vi "Config Process.vi"(8 "error in (no error)":errorcluster, 11 "View Model":T3) -> (0 "error out":errorcluster)   [LabVIEW 2017]
doc: "Configuration DB Process provide full access to the data records\nand process requests from controller\n[Covers: SD6]"
uses:
  Model/Controls/View Model.ctl
  Model/Controls/Shared Model.ctl
  Model/Controls/Views Action.ctl
  Error Handler/Controls/Error Model.ctl
  Error Handler/Controls/Error Message.ctl
  Error Handler/Controls/Error Type.ctl
  Controls/Config Model.ctl
  Controls/Config DB Message.ctl
  Controls/Config DB Command.ctl
  Controls/Config DB Overhead.ctl
  Controls/Config DB Record.ctl
  Controller/Controls/Controller Model.ctl
  Views/Vehicle Position Simulation View/Controls/Vehicle - Position.ctl
  Controller/Controls/Controller Overhead.ctl
  Controller/Controls/Controller Wash Step.ctl
  Controller/Controls/Controller State.ctl
panel:
  in  "Execute":bool
  out "Config DB Records Array":T1[](array[typedef])
  in  "DB Record":T1
  in  "DB Command":T2
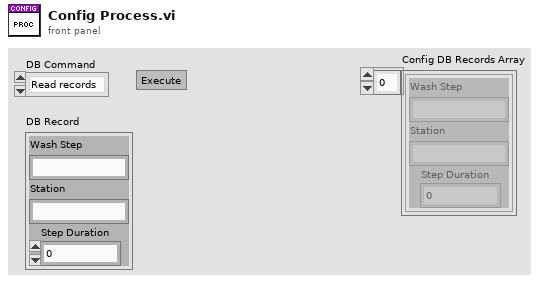
[diagram p1: front panel]
types:
  T1 = typedef "Config DB Record.ctl" = cluster{"Wash Step":string, "Station":string, "Step Duration":u32}
  T2 = typedef "Config DB Command.ctl" = enum16{"Read records", "Query timing", "Insert new data", "Update data", "Lock DB", "Unlock DB"}
  T3 = typedef "View Model.ctl" = cluster{"Shared Model":T4, "Error Model":T5, "Config Model":T6, "Controller Model":T7}
  T4 = typedef "Shared Model.ctl" = cluster{"Stop":refnum<user-event>, "Stop DVR":refnum<data-value>, "Views Action":refnum<user-event>}
  T5 = typedef "Error Model.ctl" = cluster{"Error":refnum<user-event>}
  T6 = typedef "Config Model.ctl" = cluster{"Config":refnum<user-event>, "Config DVR":refnum<data-value>}
  T7 = typedef "Controller Model.ctl" = cluster{"Position Change":refnum<user-event>, "Overhead DVR":refnum<data-value>, "Wash Cycle Start":refnum<user-event>, "Wash Step Start":refnum<user-event>, "Out Of Position":refnum<user-event>}
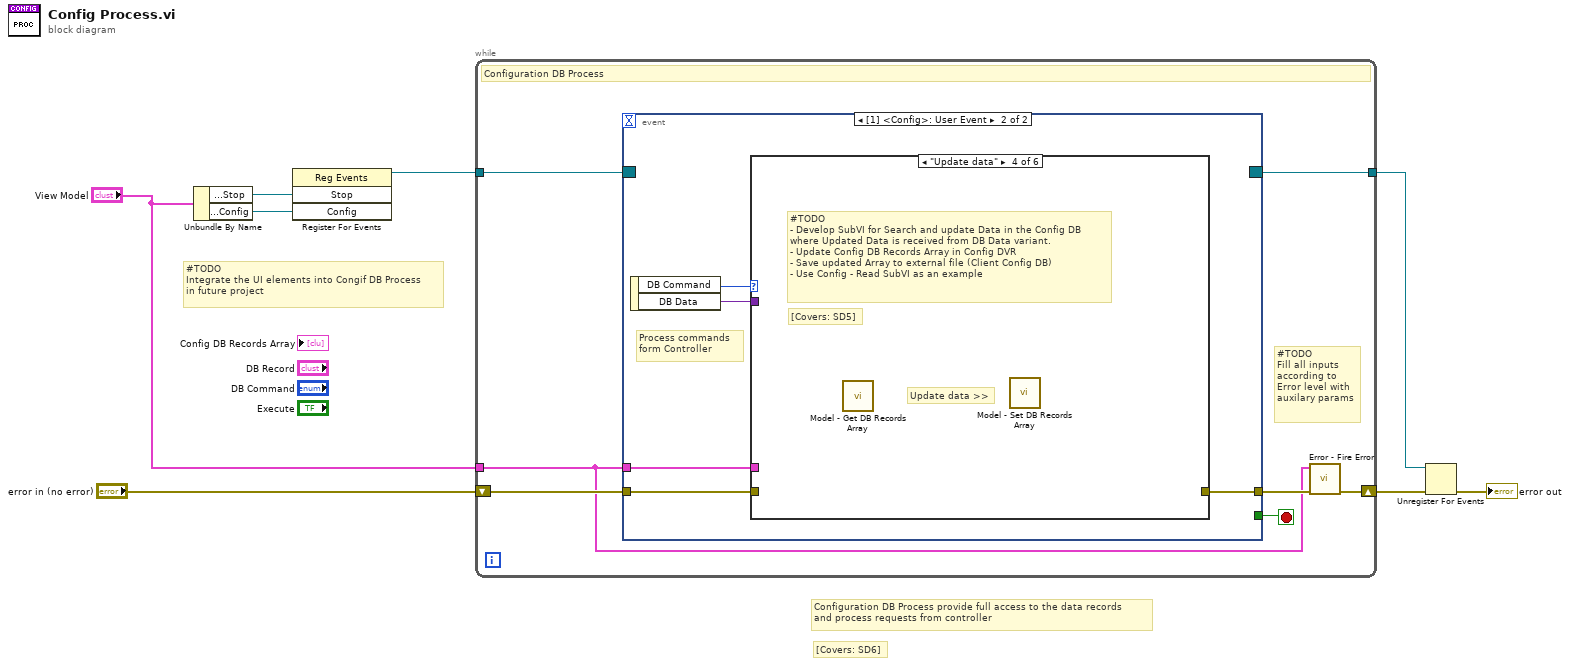
[diagram p0: block diagram]
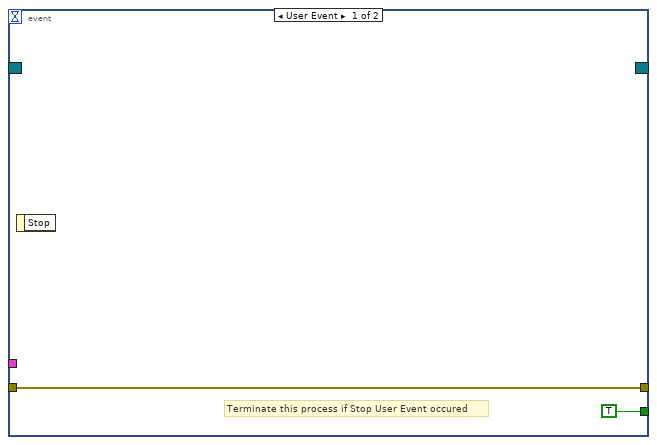
[diagram p2: hidden frame]
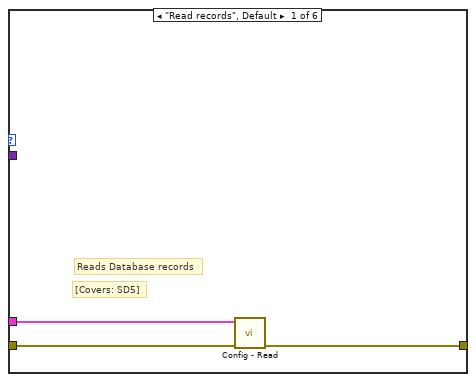
[diagram p3: hidden frame]
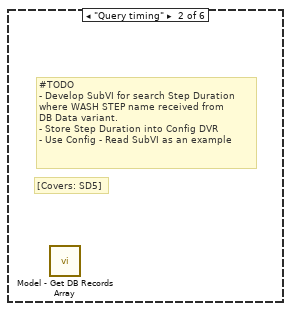
[diagram p4: hidden frame]
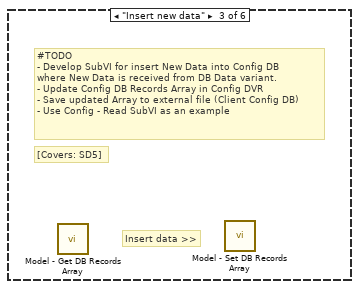
[diagram p5: hidden frame]
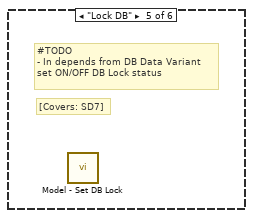
[diagram p6: hidden frame]
diagram:
  # "#TODO\nIntegrate the UI elements into Congif DB Process\nin future project"
  # "[Covers: SD6]"
  # "Configuration DB Process provide full access to the data records\nand process requests from controller"
  n1 = Unbundle By Name("View Model") -> ("Shared Model.Stop"=w8:refnum<user-event>, "Config Model.Config"=w1:refnum<user-event>)
  n2 = register-events(w8, w1) -> (reference out=w7:refnum<event-registration>)  [unwired: 2 in, 1 out]
  n3 = while {
    tunnel: w7 -> [w15]
    shift-right: [w10] -> w5
    shift-left: "error in (no error)" -> [w14]
    tunnel: [w13] -> w3
    tunnel: "View Model" -> [w9]
    stop <- w12 stop-if-true
    # "#TODO\nFill all inputs\naccording to \nError level with\nauxilary params"
    # "Configuration DB Process"
    n4 = event shown="[1] <Config>: User Event" {
      selector: w15 -> [_ _]
      dyn-events: [_ _] -> w13
      timeout: _ -> [_ _]
      tunnel: w14 -> [w17 w20]
      tunnel: [w17 w19] -> w11
      tunnel: w9 -> [_ w21]
      tunnel: [TRUE _] -> w12
      event User Event {
        # "Terminate this process if Stop User Event occured"
        n5 = event-data() -> ()  [unwired: 1 in, 1 out]
      }
      event User Event {
        # "Process commands\nform Controller"
        n6 = event-data() -> ("DB Command"=w22:T2, "DB Data"=w18:variant)  [unwired: 1 in]
        n7 = case shown="\"Update data\"" w22 {
          tunnel: w21 -> [w25 _ _ _ _ _]
          tunnel: w20 -> [w24 _ _ _ _ _]
          tunnel: [w23 _ _ _ _ _] -> w19
          tunnel: w18 -> [_ _ _ _ _ _]
          frame "Read records", Default {
            # "[Covers: SD5]"
            # "Reads Database records"
            n8 = call "Config - Read.vi"("error in (no error)"=w24, "View Model"=w25) -> ("error out"=w23:errorcluster)  [unwired: 8 in, 1 out]
          }
          frame "Query timing" {
            # "[Covers: SD5]"
            # "#TODO\n- Develop SubVI for search Step Duration\nwhere WASH STEP name received from\nDB Data variant.\n- Store Step Duration into Config DVR\n- Use Config - Read SubVI as an example"
            n9 = call "Model - Get DB Records Array.vi"() -> ()  [unwired: 9 in, 3 out]
          }
          frame "Insert new data" {
            # "Insert data >>"
            # "[Covers: SD5]"
            # "#TODO\n- Develop SubVI for insert New Data into Config DB\nwhere New Data is received from DB Data variant.\n- Update Config DB Records Array in Config DVR\n- Save updated Array to external file (Client Config DB)\n- Use Config - Read SubVI as an example"
            n10 = call "Model - Get DB Records Array.vi"() -> ()  [unwired: 9 in, 3 out]
            n11 = call "Model - Set DB Records Array.vi"() -> ()  [unwired: 10 in, 2 out]
          }
          frame "Update data" {
            # "Update data >>"
            # "[Covers: SD5]"
            # "#TODO\n- Develop SubVI for Search and update Data in the Config DB\nwhere Updated Data is received from DB Data variant.\n- Update Config DB Records Array in Config DVR\n- Save updated Array to external file (Client Config DB)\n- Use Config - Read SubVI as an example"
            n12 = call "Model - Get DB Records Array.vi"() -> ()  [unwired: 9 in, 3 out]
            n13 = call "Model - Set DB Records Array.vi"() -> ()  [unwired: 10 in, 2 out]
          }
          frame "Lock DB" {
            # "[Covers: SD7]"
            # "#TODO\n- In depends from DB Data Variant\nset ON/OFF DB Lock status"
            n14 = call "Model - Set DB Lock.vi"() -> ()  [unwired: 10 in, 2 out]
          }
          frame "Unlock DB" {
          }
        }
      }
    }
    n15 = call "Error - Fire Error.vi"("error in (no error)"=w11, "View Model"=w9) -> ("error out"=w10:errorcluster)  [unwired: 8 in, 1 out]
  }
  n16 = Unregister For Events(event registration refnum=w3, error in=w5) -> (error out=→"error out":errorcluster)
